vi "All vis.vi"   [LabVIEW 2015]
uses:
  <instrlib>/BK Precision 178XB Series/BK Precision 178XB Series.lvlib
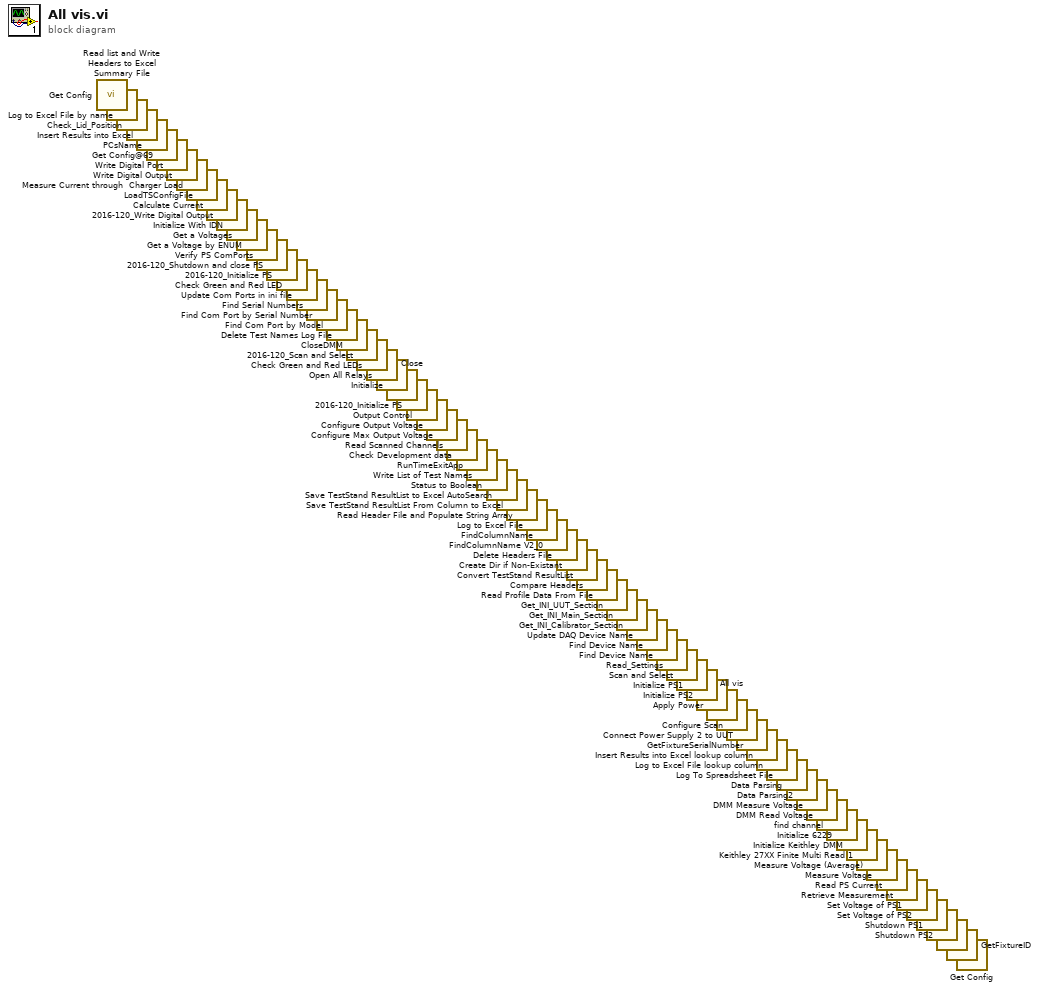
[diagram p0: block diagram]
diagram:
  n1 = call "Get Config.vi"() -> ()  [unwired: 6 in, 10 out]
  n2 = call "Read list and Write Headers to Excel Summary File.vi"() -> ()  [unwired: 8 in, 4 out]
  n3 = call "Log to Excel File by name.vi"() -> ()  [unwired: 10 in, 2 out]
  n4 = call "Check_Lid_Position.vi"() -> ()  [unwired: 10 in, 2 out]
  n5 = call "Insert Results into Excel.vi"() -> ()  [unwired: 13 in, 3 out]
  n6 = call "PCsName.vi"() -> ()  [unwired: 1 out]
  n7 = call "Get Config@69.vi"() -> ()  [unwired: 7 in, 9 out]
  n8 = call "Write Digital Port.vi"() -> ()  [unwired: 11 in, 1 out]
  n9 = call "Write Digital Output.vi"() -> ()  [unwired: 11 in, 1 out]
  n10 = call "Measure Current through  Charger Load.vi"() -> ()  [unwired: 11 in, 1 out]
  n11 = call "LoadTSConfigFile.vi"() -> ()  [unwired: 7 in, 9 out]
  n12 = call "Calculate Current.vi"() -> ()  [unwired: 11 in, 1 out]
  n13 = call "2016-120_Write Digital Output.vi"() -> ()  [unwired: 11 in, 1 out]
  n14 = call "Initialize With IDN.vi"() -> ()  [unwired: 13 in, 3 out]
  n15 = call "Get a Voltages.vi"() -> ()  [unwired: 9 in, 3 out]
  n16 = call "Get a Voltage by ENUM.vi"() -> ()  [unwired: 11 in, 1 out]
  n17 = call "Verify PS ComPorts.vi"() -> ()  [unwired: 14 in, 2 out]
  n18 = call "2016-120_Shutdown and close PS.vi"() -> ()  [unwired: 10 in, 2 out]
  n19 = call "2016-120_Initialize PS.vi"() -> ()  [unwired: 10 in, 2 out]
  n20 = call "Check Green and Red LED.vi"() -> ()  [unwired: 10 in, 2 out]
  n21 = call "Update Com Ports in ini file.vi"() -> ()  [unwired: 7 in, 9 out]
  n22 = call "Find Serial Numbers.vi"() -> ()  [unwired: 11 in, 1 out]
  n23 = call "Find Com Port by Serial Number.vi"() -> ()  [unwired: 11 in, 1 out]
  n24 = call "Find Com Port by Model.vi"() -> ()  [unwired: 11 in, 1 out]
  n25 = call "Delete Test Names Log File.vi"() -> ()  [unwired: 11 in, 1 out]
  n26 = call "CloseDMM.vi"() -> ()  [unwired: 11 in, 1 out]
  n27 = call "2016-120_Scan and Select.vi"() -> ()  [unwired: 18 in, 2 out]
  n28 = call "Check Green and Red LEDs.vi"() -> ()  [unwired: 4 in, 8 out]
  n29 = call "Open All Relays.vi"() -> ()  [unwired: 9 in, 1 out]
  n30 = call <instrlib>:"Initialize.vi"() -> ()  [unwired: 10 in, 2 out]
  n31 = call <instrlib>:"Close.vi"() -> ()  [unwired: 11 in, 1 out]
  n32 = call "2016-120_Initialize PS.vi"() -> ()  [unwired: 10 in, 2 out]
  n33 = call <instrlib>:"Output Control.vi"() -> ()  [unwired: 10 in, 2 out]
  n34 = call <instrlib>:"Configure Output Voltage.vi"() -> ()  [unwired: 14 in, 2 out]
  n35 = call <instrlib>:"Configure Max Output Voltage.vi"() -> ()  [unwired: 14 in, 2 out]
  n36 = call "Read Scanned Channels.vi"() -> ()  [unwired: 10 in, 6 out]
  n37 = call "Check Development data.vi"() -> ()  [unwired: 4 in, 2 out]
  n38 = call "RunTimeExitApp.vi"() -> ()  [unwired: 11 in, 1 out]
  n39 = call "Write List of Test Names.vi"() -> ()  [unwired: 19 in, 1 out]
  n40 = call "Status to Boolean.vi"() -> ()  [unwired: 5 in, 1 out]
  n41 = call "Save TestStand ResultList to Excel AutoSearch.vi"() -> ()  [unwired: 18 in, 2 out]
  n42 = call "Save TestStand ResultList From Column to Excel.vi"() -> ()  [unwired: 18 in, 2 out]
  n43 = call "Read Header File and Populate String Array.vi"() -> ()  [unwired: 18 in, 2 out]
  n44 = call "Log to Excel File.vi"() -> ()  [unwired: 10 in, 2 out]
  n45 = call "FindColumnName.vi"() -> ()  [unwired: 14 in, 2 out]
  n46 = call "FindColumnName V2_0.vi"() -> ()  [unwired: 14 in, 2 out]
  n47 = call "Delete Headers File.vi"() -> ()  [unwired: 11 in, 1 out]
  n48 = call "Create Dir if Non-Existant.vi"() -> ()  [unwired: 9 in, 3 out]
  n49 = call "Convert TestStand ResultList.vi"() -> ()  [unwired: 8 in, 4 out]
  n50 = call "Compare Headers.vi"() -> ()  [unwired: 19 in, 1 out]
  n51 = call "Read Profile Data From File.vi"() -> ()  [unwired: 14 in, 2 out]
  n52 = call "Get_INI_UUT_Section.vi"() -> ()  [unwired: 6 in, 6 out]
  n53 = call "Get_INI_Main_Section.vi"() -> ()  [unwired: 5 in, 4 out]
  n54 = call "Get_INI_Calibrator_Section.vi"() -> ()  [unwired: 8 in, 2 out]
  n55 = call "Update DAQ Device Name.vi"() -> ()  [unwired: 11 in, 1 out]
  n56 = call "Find Device Name.vi"() -> ()  [unwired: 11 in, 1 out]
  n57 = call "Find Device Name.vi"() -> ()  [unwired: 11 in, 1 out]
  n58 = call "Read_Settings.vi"() -> ()  [unwired: 12 in]
  n59 = call "Scan and Select.vi"() -> ()  [unwired: 18 in, 2 out]
  n60 = call "Initialize PS1.vi"() -> ()  [unwired: 10 in, 2 out]
  n61 = call "Initialize PS2.vi"() -> ()  [unwired: 10 in, 2 out]
  n62 = call "Apply Power.vi"() -> ()  [unwired: 10 in, 2 out]
  n63 = call "All vis.vi"() -> ()  [unwired: 12 in]
  n64 = call "Configure Scan.vi"() -> ()  [unwired: 10 in, 2 out]
  n65 = call "Connect Power Supply 2 to UUT.vi"() -> ()  [unwired: 12 in]
  n66 = call "GetFixtureSerialNumber.vi"() -> ()  [unwired: 8 in, 3 out]
  n67 = call "Insert Results into Excel lookup column.vi"() -> ()  [unwired: 13 in, 3 out]
  n68 = call "Log to Excel File lookup column.vi"() -> ()  [unwired: 10 in, 2 out]
  n69 = call "Log To Spreadsheet File.vi"() -> ()  [unwired: 10 in, 2 out]
  n70 = call "Data Parsing.vi"() -> ()  [unwired: 12 in, 4 out]
  n71 = call "Data Parsing2.vi"() -> ()  [unwired: 12 in, 4 out]
  n72 = call "DMM Measure Voltage.vi"() -> ()  [unwired: 9 in, 3 out]
  n73 = call "DMM Read Voltage.vi"() -> ()  [unwired: 9 in, 3 out]
  n74 = call "find channel.vi"() -> ()  [unwired: 11 in, 1 out]
  n75 = call "Initialize 6229.vi"() -> ()  [unwired: 11 in, 1 out]
  n76 = call "Initialize Keithley DMM.vi"() -> ()  [unwired: 10 in, 2 out]
  n77 = call "Keithley 27XX Finite Multi Read 1.vi"() -> ()  [unwired: 14 in, 2 out]
  n78 = call "Measure Voltage (Average).vi"() -> ()  [unwired: 9 in, 3 out]
  n79 = call "Measure Voltage.vi"() -> ()  [unwired: 9 in, 3 out]
  n80 = call "Read PS Current.vi"() -> ()  [unwired: 10 in, 2 out]
  n81 = call "Retrieve Measurement .vi"() -> ()  [unwired: 11 in, 1 out]
  n82 = call "Set Voltage of PS1.vi"() -> ()  [unwired: 11 in, 1 out]
  n83 = call "Set Voltage of PS2.vi"() -> ()  [unwired: 11 in, 1 out]
  n84 = call "Shutdown PS1.vi"() -> ()  [unwired: 11 in, 1 out]
  n85 = call "Shutdown PS2.vi"() -> ()  [unwired: 11 in, 1 out]
  n86 = call "GetFixtureID.vi"() -> ()  [unwired: 9 in, 3 out]
  n87 = call "Get Config.vi"() -> ()  [unwired: 6 in, 10 out]
